vi "2023 Teleop Arm with Setpoint Control.vi"(3 "error in (no error)":errorcluster, 4 "Joystick Command":dbl, 5 "MotorControlDevRef":T1) -> (0 "error out":errorcluster, 1 "Commanded\nSet Output":dbl, 2 "MotorControlOutput":T1={"DeviceStatus"={"status"=FALSE, "code"=0, "source"=""}, "Type"=enum."PWM", "PWM"={"PWM Channel"=enum."Invalid", "DeadBand"={"Name"="", "maxPositivePwm"=0, "minPositivePwm"=0, "centerPwm"=0, "maxNegativePwm"=0, "minNegativePwm"=0, "angularRange"=0}}, "CAN"={"Device Number"=0, "SetOutput VI Ref"=variant(refnum<vi> refnum), "GetOutput VI Ref"=variant(refnum<vi> refnum), "Enable VI Ref"=variant(refnum<vi> refnum), "Disable VI Ref"=variant(refnum<vi> refnum), "Data"=variant}, "Invert"=FALSE, "DIO PWM"={"PWM \"Enable\" Channel"=enum."Invalid", "DIOChannel"=enum."Invalid", "PWM Rate"=0.0}})   [LabVIEW 2020]
doc: "This takes a value from a joystick, applies a deadband to the value and then multiples the value by 0.2 to get the value to add to the current setpoint."
uses:
  <vilib>/Rock Robotics/WPI/MotorControl/WPI_MotorControlDeviceRef.ctl
  <vilib>/Rock Robotics/WPI/MotorControl/WPI_MotorControlType.ctl
  <vilib>/Rock Robotics/SystemInterfaces/DIO/FPGA_DIOPWMChannel.ctl
  <vilib>/Rock Robotics/WPI/PWM/WPI_PWMDeadband.ctl
  <vilib>/Rock Robotics/SystemInterfaces/DIO/FPGA_DIOChannel.ctl
  <vilib>/Rock Robotics/WPI/ThirdParty/REV Robotics/REVLib/Typedef/Spark MAX Control Type.ctl
  2022 Robot Global Data.vi
  <vilib>/Rock Robotics/Network Tables/NT Write Number.vi
  2023 Robot Global Data.vi
panel:
  out "Error\n(armSetpoint -\n armPosition)":dbl
  out "Premove\nSensor Position":dbl
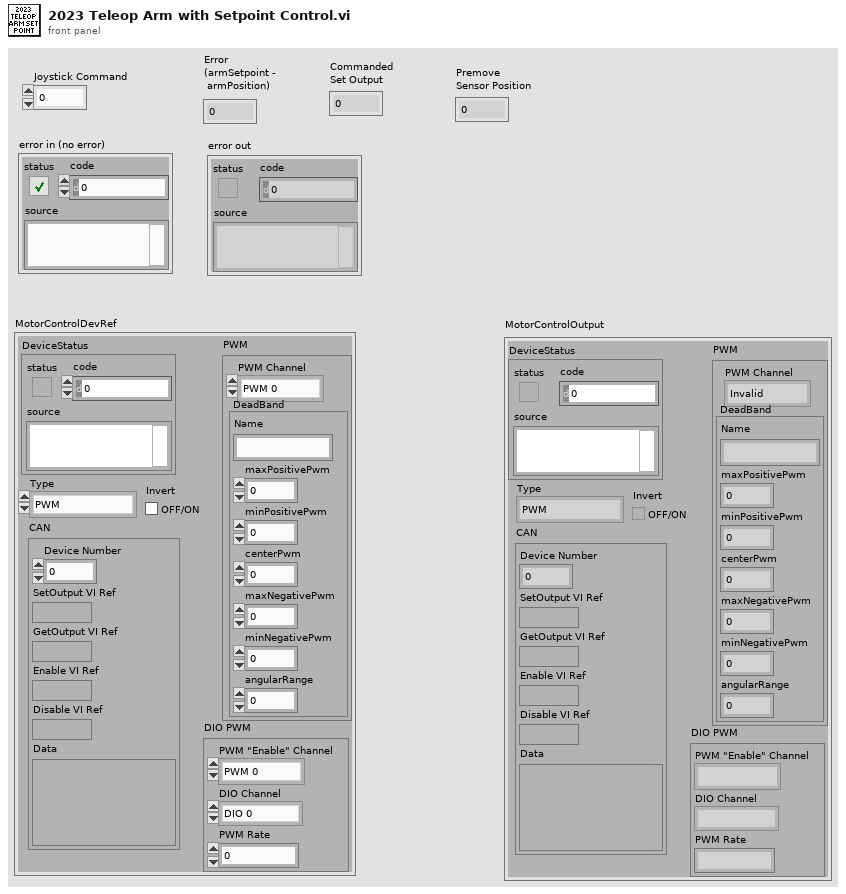
[diagram p1: front panel]
types:
  T1 = typedef "WPI_MotorControlDeviceRef.ctl" = cluster{"DeviceStatus":errorcluster, "Type":T2, "PWM":cluster{"PWM Channel":T3, "DeadBand":T4}, "CAN":cluster{"Device Number":u8, "SetOutput VI Ref":variant, "GetOutput VI Ref":variant, "Enable VI Ref":variant, "Disable VI Ref":variant, "Data":variant}, "Invert":bool, "DIO PWM":cluster{"PWM \"Enable\" Channel":T3, "DIOChannel":T5, "PWM Rate":dbl}}
  T2 = typedef "WPI_MotorControlType.ctl" = enum16{"PWM", "CAN", "DIO PWM"}
  T3 = typedef "FPGA_DIOPWMChannel.ctl" = enum8{"PWM 0", "PWM 1", "PWM 2", "PWM 3", "PWM 4", "PWM 5", "PWM 6", "PWM 7", "PWM 8", "PWM 9", "PWM MXP 0", "PWM MXP 1", "PWM MXP 2", "PWM MXP 3", "PWM MXP 4", "PWM MXP 5", "PWM MXP 6", "PWM MXP 7", "PWM MXP 8", "PWM MXP 9", "Invalid"}
  T4 = typedef "WPI_PWMDeadband.ctl" = cluster{"Name":string, "maxPositivePwm":i32, "minPositivePwm":i32, "centerPwm":i32, "maxNegativePwm":i32, "minNegativePwm":i32, "angularRange":u16}
  T5 = typedef "FPGA_DIOChannel.ctl" = enum8{"DIO 0", "DIO 1", "DIO 2", "DIO 3", "DIO 4", "DIO 5", "DIO 6", "DIO 7", "DIO 8", "DIO 9", "DIO MXP 0", "DIO MXP 1", "DIO MXP 2", "DIO MXP 3", "DIO MXP 4", "DIO MXP 5", "DIO MXP 6", "DIO MXP 7", "DIO MXP 8", "DIO MXP 9", "DIO MXP 10", "DIO MXP 11", "DIO MXP 12", "DIO MXP 13", "DIO MXP 14", "DIO MXP 15", "SPI Port CS1", "SPI Port CS2", "SPI Port CS3", "SPI Port MISO", "SPI Port MOSI", "Invalid"}
  T6 = typedef "Spark MAX Control Type.ctl" = enum16{"Percent VBus", "Voltage", "Velocity", "Position", "Smart Motion", "Current", "Smart Velocity"}
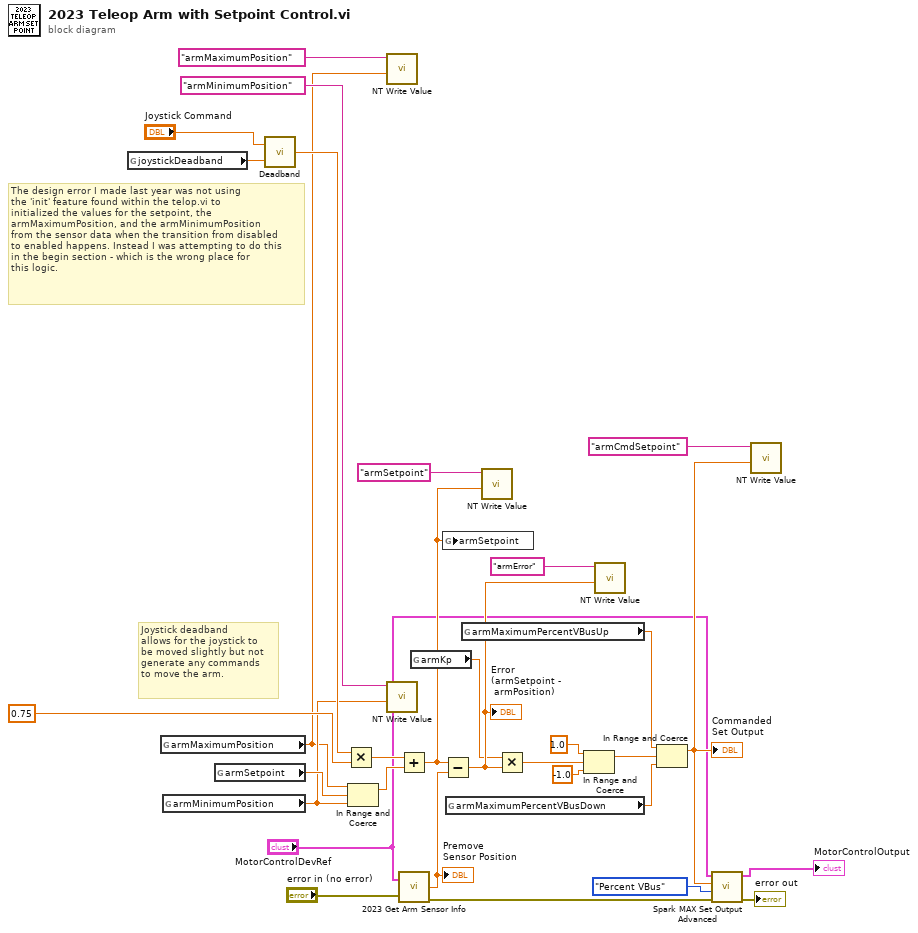
[diagram p0: block diagram]
diagram:
  # "The design error I made last year was not using\nthe 'init' feature found within the telop.vi to \ninitialized the values for the setpoint, the\narmMaximumPosition, and the armMinimumPosition\nfrom the sensor data when the transition from disabled\nto enabled happens. Instead I was attempting to do this\nin the begin section - which is the wrong place for\nthis logic."
  # "Joystick deadband\nallows for the joystick to\nbe moved slightly but not\ngenerate any commands\nto move the arm."
  n1 = global read "2022 Robot Global Data.vi" "joystickDeadband"() -> (w16:dbl)
  n2 = global read "2022 Robot Global Data.vi" "armMaximumPosition"() -> (w4:dbl)
  n3 = global read "2022 Robot Global Data.vi" "armMinimumPosition"() -> (w5:dbl)
  n4 = global read "2022 Robot Global Data.vi" "armSetpoint"() -> (w22:dbl)
  n5 = call "Deadband.vi"("Limit"=w16, "Input"="Joystick Command") -> ("Output"=w21:dbl)
  n6 = Multiply(x=w21, y=0.75) -> (x*y=w23:dbl)
  n7 = In Range and Coerce(upper limit=w4, x=w22, lower limit=w5) -> (coerced(x)=w24:dbl)  [unwired: 1 out]
  n8 = call-poly <vilib>:"NT Write Value.vi"("value"=w4, "name"="armMaximumPosition") -> ()  [unwired: 9 in, 1 out]
  n9 = call-poly <vilib>:"NT Write Value.vi"("value"=w5, "name"="armMinimumPosition") -> ()  [unwired: 9 in, 1 out]
  n10 = Add(x=w23, y=w24) -> (x+y=w10:dbl)
  n11 = call "2023 Get Arm Sensor Info.vi"("error in (no error)"="error in (no error)", "MotorControlDevRef"="MotorControlDevRef") -> ("error out"=w14:errorcluster, "Sensor Position"=w15:dbl)  [unwired: 3 out]
  "Premove\nSensor Position" <- w15
  n12 = global read "2023 Robot Global Data.vi" "armKp"() -> (w3:dbl)
  n13 = global write "2022 Robot Global Data.vi" "armSetpoint"(w10) -> ()
  n14 = Subtract(x=w10, y=w15) -> (x-y=w8:dbl)
  "Error\n(armSetpoint -\n armPosition)" <- w8
  n15 = global read "2022 Robot Global Data.vi" "armMaximumPercentVBusDown"() -> (w17:dbl)
  n16 = global read "2022 Robot Global Data.vi" "armMaximumPercentVBusUp"() -> (w30:dbl)
  n17 = call-poly <vilib>:"NT Write Value.vi"("value"=w10, "name"="armSetpoint") -> ()  [unwired: 9 in, 1 out]
  n18 = Multiply(x=w3, y=w8) -> (x*y=w27:dbl)
  n19 = In Range and Coerce(upper limit=1.0, x=w27, lower limit=-1.0) -> (coerced(x)=w28:dbl)  [unwired: 1 out]
  n20 = call-poly <vilib>:"NT Write Value.vi"("value"=w8, "name"="armError") -> ()  [unwired: 9 in, 1 out]
  n21 = In Range and Coerce(upper limit=w30, x=w28, lower limit=w17) -> (coerced(x)=w12:dbl)  [unwired: 1 out]
  "Commanded\nSet Output" <- w12
  n22 = call <vilib>:"Spark MAX Set Output Advanced.vi"("error in (no error)"=w14, "Control Mode"=Spark_MAX_Control_Type."Percent VBus", "Setpoint"=w12, "MotorControlDevRef"="MotorControlDevRef") -> ("error out"=→"error out":errorcluster, "MotorControlDevRef"=→"MotorControlOutput":T1)  [unwired: 6 in]
  n23 = call-poly <vilib>:"NT Write Value.vi"("value"=w12, "name"="armCmdSetpoint") -> ()  [unwired: 9 in, 1 out]
